vi "ColorSelector.vi"() -> (1 "颜色":u32(colorbox))   [LabVIEW 2015]
panel:
  out "灰度选择":picture
  out "全彩选择":picture
  out "B:":u8
  out "G:":u8
  out "R:":u8
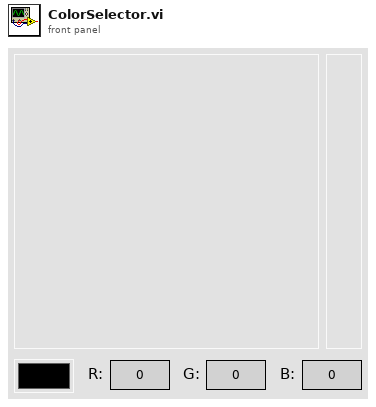
[diagram p1: front panel]
types:
  T1 = cluster{"图片宽1":i16, "image1":u8[], "图片宽2":i16, "image2":u8[]}
  T2 = typedef "imagedata.ctl" = cluster{"image type":i32, "image depth":i32, "image":u8[], "mask":u8[], "colors":u32[], "Rectangle":cluster{"left":i16, "top":i16, "right":i16, "bottom":i16}}
  T3 = typedef "LVMouseTypeDef.ctl" = cluster{"Mouse Position":cluster{"X":i32, "Y":i32}, "Mouse Modifiers":cluster{"Button Down":bool, "Shift Mod":bool, "Menu Mod":bool, "Option Mod":bool}}
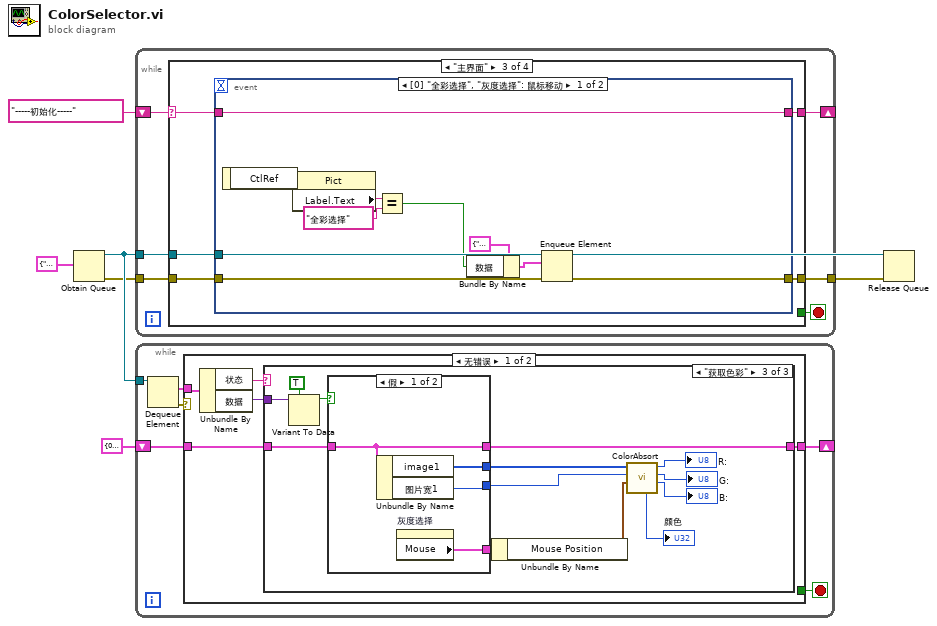
[diagram p0: block diagram]
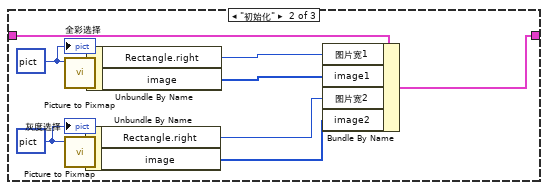
[diagram p3: hidden frame]
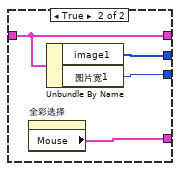
[diagram p4: hidden frame]
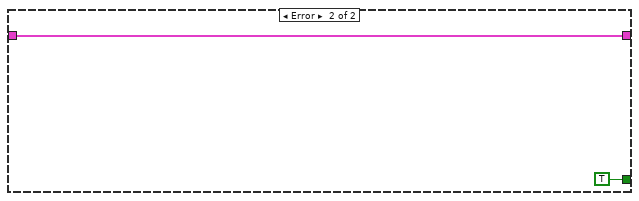
[diagram p5: hidden frame]
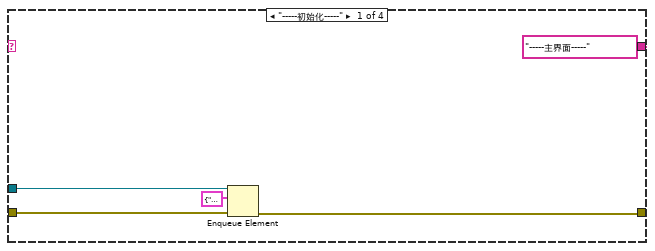
[diagram p6: hidden frame]
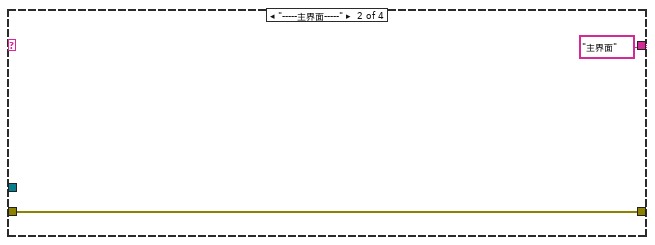
[diagram p7: hidden frame]
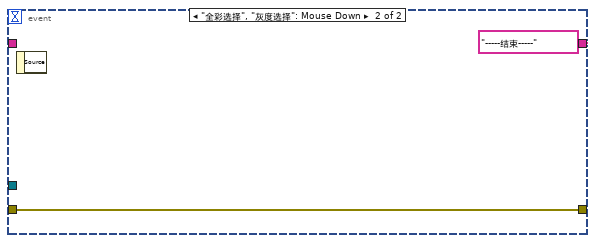
[diagram p8: hidden frame]
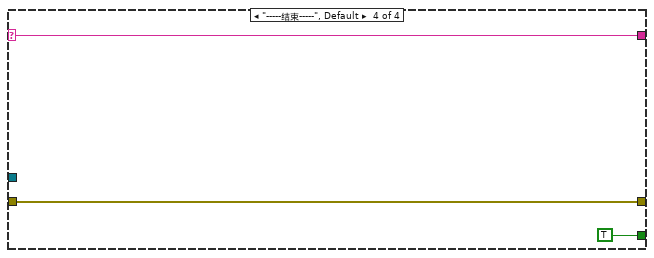
[diagram p9: hidden frame]
diagram:
  n1 = Obtain Queue(element data type=cluster{"状态":string, "数据":variant} {"状态"="", "数据"=variant}) -> (queue out=w6:refnum<queue>, error out=w4:errorcluster)  [unwired: 4 in, 1 out]
  n2 = while {
    tunnel: w6 -> [w12]
    shift-right: [w11] -> _
    shift-left: "-----初始化-----" -> [w10]
    tunnel: w4 -> [w8]
    tunnel: [w7] -> w3
    stop <- w9 stop-if-true
    n3 = case shown="\"主界面\"" w10 {
      selector: w10 -> [_ _ w20 w38]
      tunnel: w12 -> [w16 _ w24 _]
      tunnel: w8 -> [w15 w18 w23 w39]
      tunnel: [w14 w18 w22 w39] -> w7
      tunnel: ["-----主界面-----" "主界面" w21 w38] -> w11
      tunnel: [_ _ _ TRUE] -> w9
      frame "-----初始化-----" {
        n4 = Enqueue Element(queue=w16, element=cluster{"状态":string, "数据":variant} {"状态"="初始化", "数据"=variant} ("元素"), error in (no error)=w15) -> (error out=w14:errorcluster)  [unwired: 1 in, 2 out]
      }
      frame "-----主界面-----" {
      }
      frame "主界面" {
        n5 = event shown="[0] \"全彩选择\", \"灰度选择\": 鼠标移动" {
          selector: _ -> [_ _]
          dyn-events: _ -> [_ _]
          timeout: _ -> [_ _]
          tunnel: w24 -> [w34 _]
          tunnel: w23 -> [w33 w36]
          tunnel: [w32 w36] -> w22
          tunnel: [w31 "-----结束-----"] -> w21
          tunnel: w20 -> [w31 _]
          event "全彩选择", "灰度选择": Mouse Move {
            n6 = event-data() -> ("CtlRef"=w29:refnum<vi>)  [unwired: 1 in]
            n7 = property class="Pict"(reference=w29) -> ("Label.Text"=w28:string)  [unwired: 1 in, 2 out]
            n8 = Equal?(x=w28, y="全彩选择") -> (x = y?=w25:bool)
            n9 = Bundle By Name(cluster=cluster{"状态":string, "数据":variant} {"状态"="获取色彩", "数据"=variant} ("元素"), "数据"=w25) -> (w26:cluster{"状态":string, "数据":variant})
            n10 = Enqueue Element(queue=w34, element=w26, error in (no error)=w33) -> (error out=w32:errorcluster)  [unwired: 1 in, 2 out]
          }
          event "全彩选择", "灰度选择": Mouse Down {
            n11 = event-data() -> ()  [unwired: 1 in, 1 out]
          }
        }
      }
      frame "-----结束-----", Default {
      }
    }
  }
  n12 = while {
    tunnel: w6 -> [w45]
    shift-right: [w41] -> _
    shift-left: T1 {"图片宽1"=0, "image1"=[], "图片宽2"=0, "image2"=[]} -> [w40]
    stop <- w42 stop-if-true
    n13 = Dequeue Element(queue=w45) -> (element=w43:cluster{"状态":string, "数据":variant}, error out=w44:errorcluster)  [unwired: 2 in, 2 out]
    n14 = case shown="无错误" w44 {
      tunnel: w43 -> [w48 _]
      tunnel: [_ TRUE] -> w42
      tunnel: [w50 w83] -> w41
      tunnel: w40 -> [w49 w83]
      frame No Error {
        n15 = Unbundle By Name(w48) -> ("状态"=w47:string, "数据"=w46:variant)
        n16 = case shown="\"获取色彩\"" w47 {
          tunnel: [w51 w52 w65] -> w50
          tunnel: w49 -> [w51 w57 w64]
          tunnel: w46 -> [_ _ w68]
          frame "假", Default {
          }
          frame "初始化" {
            w60 = picture bytes[28641] ("二维图片2")
            w61 = picture bytes[269378] ("二维图片")
            n17 = call <vilib>:"Picture to Pixmap.vi"("picture"=w61) -> ("image data"=w58:T2)  [unwired: 9 in, 1 out]
            n18 = call <vilib>:"Picture to Pixmap.vi"("picture"=w60) -> ("image data"=w59:T2)  [unwired: 9 in, 1 out]
            n19 = Unbundle By Name(w59) -> ("Rectangle.right"=w54:i16, "image"=w53:u8[])
            n20 = Unbundle By Name(w58) -> ("Rectangle.right"=w56:i16, "image"=w55:u8[])
            n21 = Bundle By Name(cluster=w57, "图片宽1"=w56, "image1"=w55, "图片宽2"=w54, "image2"=w53) -> (w52:T1)
            "全彩选择" <- w61
            "灰度选择" <- w60
          }
          frame "获取色彩" {
            n22 = Variant To Data(type=TRUE, Variant=w68) -> (data=w66:bool)  [unwired: 1 in, 1 out]
            n23 = case shown="假" w66 {
              tunnel: [w75 w82] -> w69
              tunnel: [w76 w81] -> w65
              tunnel: w64 -> [w76 w81]
              tunnel: [w78 w80] -> w63
              tunnel: [w77 w79] -> w62
              frame False {
                n24 = Unbundle By Name(w76) -> ("image1"=w78:u8[], "图片宽1"=w77:i16)
                n25 = property on="灰度选择" class="Pict"() -> ("Mouse"=w75:T3)  [unwired: 2 in, 2 out]
              }
              frame True {
                n26 = property on="全彩选择" class="Pict"() -> ("Mouse"=w82:T3)  [unwired: 2 in, 2 out]
                n27 = Unbundle By Name(w81) -> ("image1"=w80:u8[], "图片宽1"=w79:i16)
              }
            }
            n28 = Unbundle By Name(w69) -> ("Mouse Position"=w70:cluster{"X":i32, "Y":i32})
            n29 = call "ColorAbsort.vi"("位置"=w70, "图片宽"=w62, "image"=w63) -> ("B"=→"B:":u8, "G"=→"G:":u8, "R"=→"R:":u8, "颜色盒"=→"颜色":u32)  [unwired: 4 in, 1 out]
          }
        }
      }
      frame Error {
      }
    }
  }
  n30 = Release Queue(queue=w6, error in (no error)=w3) -> ()  [unwired: 1 in, 3 out]
